vi "set page.vi"(0 "VISA in":refnum<visa-resource-name>, 1 "Location Cluster in":T1, 2 "num pages":i32, 3 "set page":i32, 5 "error in":errorcluster) -> (14 "VISA out":refnum<visa-resource-name>, 15 "Location Cluster out":T1, 19 "error out":errorcluster)   [LabVIEW 2018]
uses:
  location cluster.ctl
  CAEN globals.vi
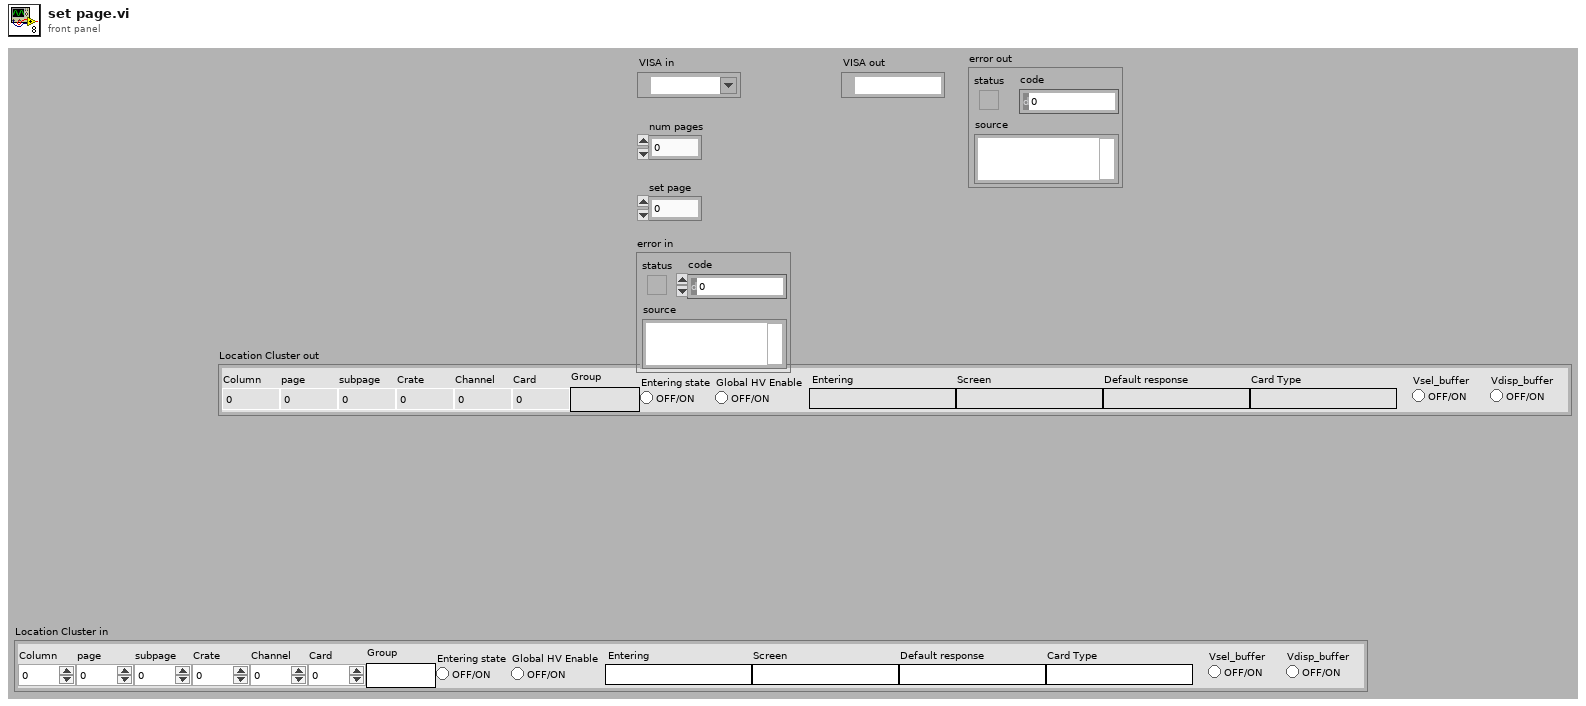
[diagram p1: front panel]
types:
  T1 = typedef "location cluster.ctl" = cluster{"Column":i32, "Card Type":string, "Channel":i32, "Card":i32, "Default response":string, "Entering":string, "Entering state":bool, "subpage":i32, "page":i32, "Crate":i32, "Screen":string, "Group":string, "Global HV Enable":bool, "Vsel_buffer":bool, "Vdisp_buffer":bool}
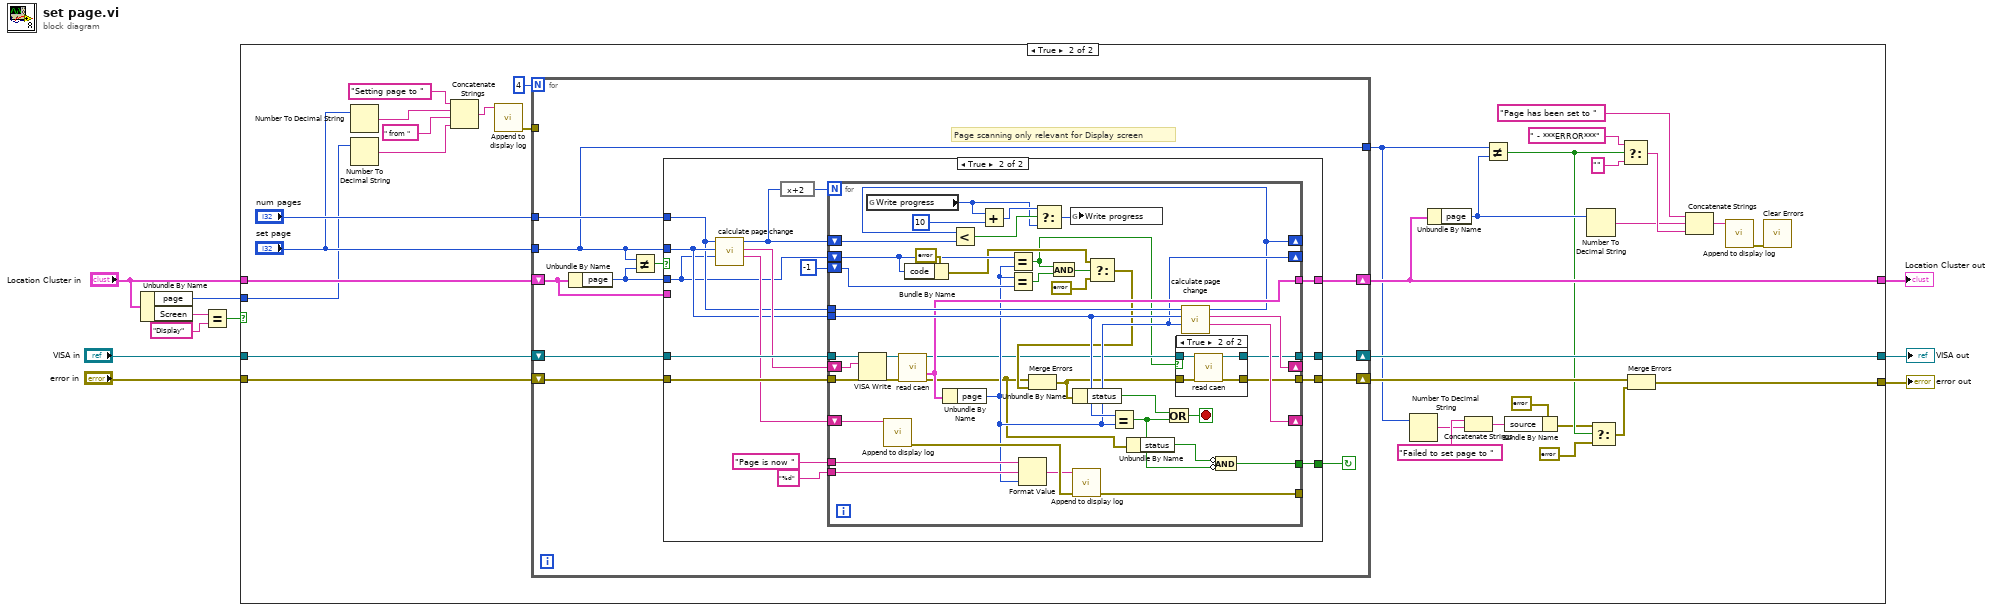
[diagram p0: block diagram]
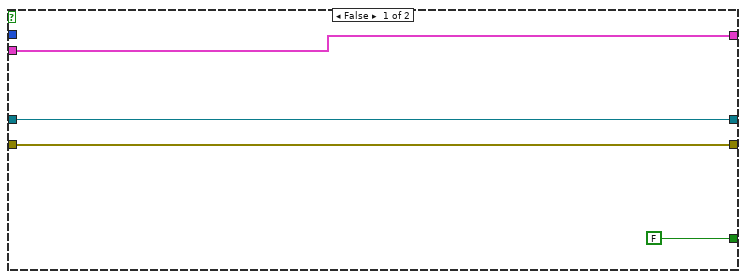
[diagram p3: hidden frame]
diagram:
  n1 = Unbundle By Name("Location Cluster in") -> ("page"=w6:i32, "Screen"=w2:string)
  n2 = Equal?(x=w2, y="Display" ("x")) -> (x = y?=w1:bool)
  n3 = case shown="True" w1 {
    tunnel: [w12 w47] -> w10
    tunnel: "error in" -> [w13 w45]
    tunnel: "VISA in" -> [w12 w44]
    tunnel: "Location Cluster in" -> [w11 w42]
    tunnel: w6 -> [_ w35]
    tunnel: [w11 w25] -> w5
    tunnel: [w13 w23] -> w4
    frame False {
    }
    frame True {
      n4 = Number To Decimal String(number="set page") -> (decimal integer string=w39:string)  [unwired: 1 in]
      n5 = Number To Decimal String(number=w35) -> (decimal integer string=w41:string)  [unwired: 1 in]
      n6 = Concatenate Strings("Setting page to " ("string"), w39, " from " ("string"), w41) -> (w37:string)
      n7 = call "Append to display log.vi"("string"=w37) -> ("error out"=w34:errorcluster)  [unwired: 10 in]
      n8 = for {
        N: 4 -> [_]
        tunnel: "num pages" -> [w55]
        tunnel: "set page" -> [w49]
        shift-right: [w51] -> w25
        shift-left: w42 -> [w56]
        shift-right: [w58] -> w24
        shift-left: w45 -> [w54]
        shift-right: [w57] -> w47
        shift-left: w44 -> [w53]
        tunnel: w34 -> [_]
        tunnel: [w49] -> w14
        stop <- w50 continue-if-true
        # "Page scanning only relevant for Display screen"
        n9 = Unbundle By Name(w56) -> ("page"=w52:i32)
        n10 = Not Equal?(x=w49, y=w52) -> (x != y?=w48:bool)
        n11 = case shown="True" w48 {
          tunnel: w53 -> [w61 w78]
          tunnel: w54 -> [w60 w77]
          tunnel: w52 -> [_ w65]
          tunnel: w49 -> [_ w68]
          tunnel: w55 -> [_ w67]
          tunnel: [w61 w75] -> w57
          tunnel: [w60 w74] -> w58
          tunnel: w56 -> [w62 _]
          tunnel: [w62 w69] -> w51
          tunnel: [FALSE w66] -> w50
          frame False {
          }
          frame True {
            n12 = call "calculate page change.vi"("current page"=w65, "set page"=w68, "num pages"=w67) -> ("action"=w71:string, "keystroke"=w76:string, "page changes rqd"=w64:i32)  [unwired: 6 in]
            n13 = expression code="x+2"(w64) -> (w70:i32)
            n14 = for {
              N: w70 -> [_]
              tunnel: w78 -> [w121]
              tunnel: w77 -> [w120]
              tunnel: [w82] -> w75
              tunnel: [w85] -> w74
              tunnel: "Page is now " ("set Screen") -> [w113]
              tunnel: "%d" ("set Screen") -> [w112]
              tunnel: [w111] -> _
              tunnel: [w101] -> w69
              tunnel: w68 -> [w108]
              shift-right: [w106] -> _
              shift-left: w76 -> [w119]
              tunnel: w67 -> [w109]
              shift-right: [w107] -> _
              shift-left: w71 -> [w116]
              tunnel: [w104] -> w66
              shift-right: [w99] -> _
              shift-left: w65 -> [w87]
              shift-left: -1 ("page") -> [w100]
              shift-right: [w90] -> _
              shift-left: w64 -> [w95]
              stop <- w110 stop-if-true
              n15 = VISA Write(VISA resource name=w121, write buffer=w119, error in (no error)=w120) -> (VISA resource name out=w118:refnum<visa-resource-name>, error out=w117:errorcluster)  [unwired: 1 out]
              n16 = global read "CAEN globals.vi" "Write progress"() -> (w92:u8)
              n17 = call "Append to display log.vi"("string"=w116) -> ("error out"=w115:errorcluster)  [unwired: 10 in]
              n18 = call "read caen.vi"("VISA in"=w118, "error in"=w117) -> ("VISA out"=w83:refnum<visa-resource-name>, "Location Cluster"=w101:T1, "error out"=w79:errorcluster)  [unwired: 8 in, 3 out]
              n19 = Bundle By Name(cluster=errorcluster {"status"=TRUE, "code"=0, "source"="Page changing failed"} ("error in"), "code"=w87) -> (w86:errorcluster)
              n20 = Unbundle By Name(w101) -> ("page"=w99:i32)
              n21 = Add(x=w92, y=u8 10) -> (x+y=w93:u8)
              n22 = Equal?(x=w87, y=w99) -> (x = y?=w81:bool)
              n23 = Equal?(x=w99, y=w100) -> (x = y?=w98:bool)
              n24 = Format Value(string ("")=w113, format string=w112, value (0)=w99) -> (output string=w114:string)
              n25 = And(x=w81, y=w98) -> (x .and. y?=w97:bool)
              n26 = call "Append to display log.vi"("error in"=w115, "string"=w114) -> ("error out"=w111:errorcluster)  [unwired: 9 in]
              n27 = Select(t=w86, s=w97, f=errorcluster {"status"=FALSE, "code"=0, "source"=""} ("error in")) -> (s? t:f=w96:errorcluster)
              n28 = Merge Errors(w79, w96) -> (w84:errorcluster)
              n29 = Unbundle By Name(w84) -> ("status"=w105:bool)
              n30 = Equal?(x=w108, y=w99) -> (x = y?=w103:bool)
              n31 = Unbundle By Name(w79) -> ("status"=w80:bool)
              n32 = Or(x=w105, y=w103) -> (x .or. y?=w110:bool)
              n33 = case shown="True" w81 {
                tunnel: [w122 w127] -> w85
                tunnel: w84 -> [w122 w126]
                tunnel: w83 -> [w123 w125]
                tunnel: [w123 w124] -> w82
                frame False {
                }
                frame True {
                  n34 = call "read caen.vi"("VISA in"=w125, "error in"=w126) -> ("VISA out"=w124:refnum<visa-resource-name>, "error out"=w127:errorcluster)  [unwired: 8 in, 4 out]
                }
              }
              n35 = call "calculate page change.vi"("current page"=w99, "set page"=w108, "num pages"=w109) -> ("action"=w107:string, "keystroke"=w106:string, "page changes rqd"=w90:i32)  [unwired: 6 in]
              n36 = Less?(x=w90, y=w95) -> (x < y?=w94:bool)
              n37 = Select(t=w93, s=w94, f=w92) -> (s? t:f=w91:u8)
              n38 = global write "CAEN globals.vi" "Write progress"(w91) -> ()
              n39 = Compound Arithmetic op=AND(invert w80, invert w103) -> (w104:bool)
            }
          }
        }
      }
      n40 = Number To Decimal String(number=w14) -> (decimal integer string=w15:string)  [unwired: 1 in]
      n41 = Unbundle By Name(w25) -> ("page"=w30:i32)
      n42 = Concatenate Strings("Failed to set page to " ("string"), w15) -> (w17:string)
      n43 = Not Equal?(x=w14, y=w30) -> (x != y?=w21:bool)
      n44 = Bundle By Name(cluster=errorcluster {"status"=TRUE, "code"=0, "source"=""} ("error in"), "source"=w17) -> (w18:errorcluster)
      n45 = Number To Decimal String(number=w30) -> (decimal integer string=w28:string)  [unwired: 1 in]
      n46 = Select(t=w18, s=w21, f=errorcluster {"status"=FALSE, "code"=0, "source"=""} ("error in")) -> (s? t:f=w22:errorcluster)
      n47 = Select(t=" - ***ERROR***" ("string"), s=w21, f="" ("string")) -> (s? t:f=w33:string)
      n48 = Merge Errors(w24, w22) -> (w23:errorcluster)
      n49 = Concatenate Strings("Page has been set to " ("string"), w28, w33) -> (w27:string)
      n50 = call "Append to display log.vi"("string"=w27) -> ("error out"=w29:errorcluster)  [unwired: 10 in]
      n51 = call <vilib>:"Clear Errors.vi"("error in (no error)"=w29) -> ()  [unwired: 5 in, 2 out]
    }
  }
  "Location Cluster out" <- w5
  "error out" <- w4
  "VISA out" <- w10
